vi "FreePort.vi"(8 "error in (no error)":errorcluster, 10 "Preferred Port":i64, 11 "MicronCLI in":refnum<class "MicronCLI.lvclass">) -> (0 "error out":errorcluster, 2 "Port Out":i64, 3 "MicronCLI out":refnum<class "MicronCLI.lvclass">)   [LabVIEW 2019, in "MicronCLI.lvclass"]
doc: "Find Free Port"
uses:
  MicronCLI.lvclass
  MicronCLI.lvclass/MicronCLI.ctl
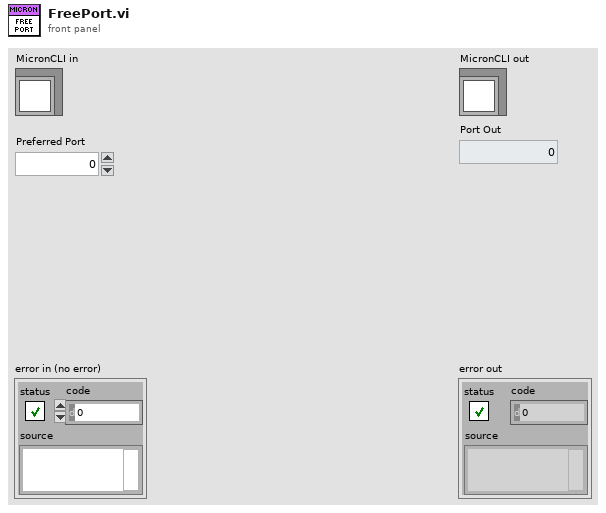
[diagram p1: front panel]
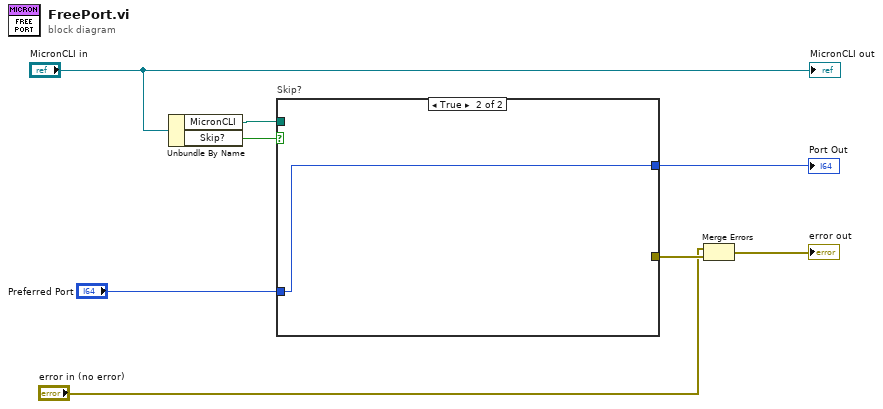
[diagram p0: block diagram]
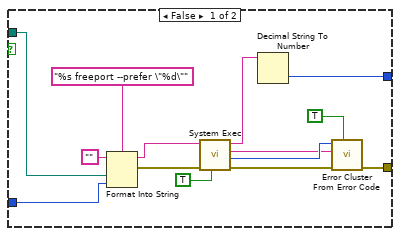
[diagram p2: hidden frame]
diagram:
  n1 = Unbundle By Name("MicronCLI in") -> ("MicronCLI"=w5:path, "Skip?"=w4:bool)
  n2 = case "Skip?" shown="True" w4 {
    tunnel: w5 -> [w19 _]
    tunnel: [w15 _] -> w8
    tunnel: "Preferred Port" -> [w11 w23]
    tunnel: [w9 w23] -> w1
    frame False {
      n3 = Format Into String(format string="%s freeport --prefer \"%d\"", initial string="", w19, w11) -> (resulting string=w17:string, error out=w21:errorcluster)  [unwired: 1 in]
      n4 = call <vilib>:"System Exec.vi"("run minimized? (F)"=TRUE, "error in (no error)"=w21, "command line"=w17) -> ("error out"=w22:errorcluster, "return code"=w14:i32, "standard error"=w13:string, "standard output"=w10:string)  [unwired: 5 in]
      n5 = Decimal String To Number(string=w10) -> (number=w9:i32)  [unwired: 2 in, 1 out]
      n6 = call <vilib>:"Error Cluster From Error Code.vi"("show call chain? (False)"=TRUE, "error in (no error)"=w22, "error message (\"\")"=w13, "error code (0)"=w14) -> ("error out"=w15:errorcluster)  [unwired: 5 in]
    }
    frame True {
    }
  }
  "Port Out" <- w1
  n7 = Merge Errors("error in (no error)", w8) -> (→"error out":errorcluster)
  "MicronCLI out" <- "MicronCLI in"
